vi "close.vi"(6 "RH?":bool, 8 "error in (no error)":errorcluster) -> (0 "error out":errorcluster)   [LabVIEW 2017]
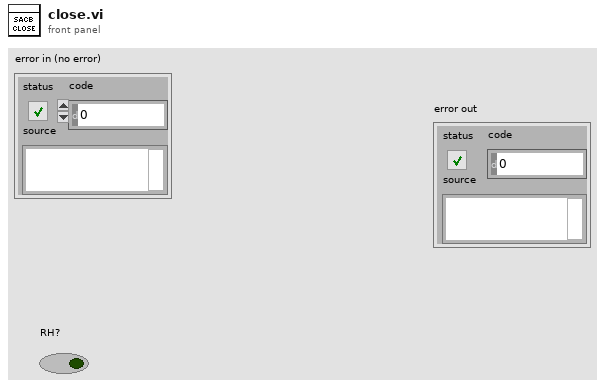
[diagram p1: front panel]
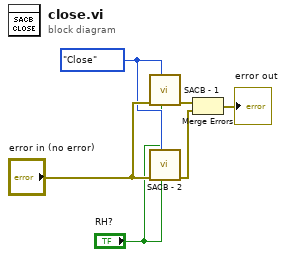
[diagram p0: block diagram]
diagram:
  w5 = enum16{"Create", "Read", "Close"}."Close" ("Command")
  n1 = call "SACB - 1.vi"("RH?"="RH?", "Command"=w5, "Error In"="error in (no error)") -> ("Error Out"=w4:errorcluster)  [unwired: 7 in, 1 out]
  n2 = call "SACB - 2.vi"("RH?"="RH?", "Command"=w5, "Error In"="error in (no error)") -> ("Error Out"=w3:errorcluster)  [unwired: 7 in, 1 out]
  n3 = Merge Errors(w4, w3) -> (→"error out":errorcluster)
